vi "DAQ_CounterTrigger_DO_AO_2DAQ.vi"(8 "error in (no error)":errorcluster) -> (0 "error out":errorcluster)   [LabVIEW 2025]
uses:
  SubVIs/State_Machine_Ctrl.ctl
  <vilib>/DAQmx/write.llb/DAQmx Write (Digital 1D Wfm NChan NSamp).vi
  <vilib>/DAQmx/write.llb/DAQmx Write (Analog 1D Wfm NChan NSamp).vi
  <vilib>/Waveform/DWDTOps.llb/DWDT Uncompress Digital.vi
  <vilib>/DAQmx/miscellaneous.llb/DAQmx Fill In Error Info.vi
  <resource>/objmgr/daqmx.rc
panel:
  in  "Z":bool=TRUE
  in  "AO Z":tag="USB-6211/ao1"
  out "AO WF":waveform(dbl)[](graph)=[{"t0"=timestamp(0 s since 1904-01-01), "dt"=0.0001, "Y"=array[9000 elements]}, {"t0"=timestamp(0 s since 1904-01-01), "dt"=0.0001, "Y"=array[9000 elements]}, {"t0"=timestamp(0 s since 1904-01-01), "dt"=0.0001, "Y"=array[9000 elements]}, {"t0"=timestamp(0 s since 1904-01-01), "dt"=0.0001, "Y"=array[9000 elements]}]
  out "DO WF":digitalwaveform[](graph)=[{"t0"=timestamp(0 s since 1904-01-01), "dt"=0.0001, "Y"={"transitions"=[], "data"=array9000x1[9000 elements]}}, {"t0"=timestamp(0 s since 1904-01-01), "dt"=0.0001, "Y"={"transitions"=[], "data"=array9000x1[9000 elements]}}, {"t0"=timestamp(0 s since 1904-01-01), "dt"=0.0001, "Y"={"transitions"=[], "data"=array9000x1[9000 elements]}}, {"t0"=timestamp(0 s since 1904-01-01), "dt"=0.0001, "Y"={"transitions"=[], "data"=array9000x1[9000 elements]}}]
  in  "Polar | ON/OFF":bool=TRUE
  in  "AO | %":dbl[](array[slide])=[9.734513274336283, 23.008849557522126, 41.5929203539823, 65.48672566371681] min=0.0 max=100.0 step=1.0 scale=0.0..100.0
  in  "AO | ON/OFF":bool[](array[boolean])=[TRUE, TRUE, TRUE, TRUE]
  in  "AO Laser":tag="USB-6363/ao0:3"
  in  "AO pockels":tag="USB-6211/ao0"
  in  "DO | ON/OFF":bool[](array[boolean])=[TRUE, TRUE, TRUE, TRUE, TRUE]
  in  "Pre-activation time (s)":dbl=0.03
  in  "Start":bool
  in  "Timing source":tag="OnboardClock"
  in  "Readout time (s)":dbl=0.02
  in  "Exposure time (s)":dbl=0.05
  in  "DO | Trigger":tag="/USB-6363/PFI12"
  in  "DO":tag="USB-6363/port0/line0:4"
  in  "Counter":tag="USB-6363/ctr0"
  in  "Stop":bool
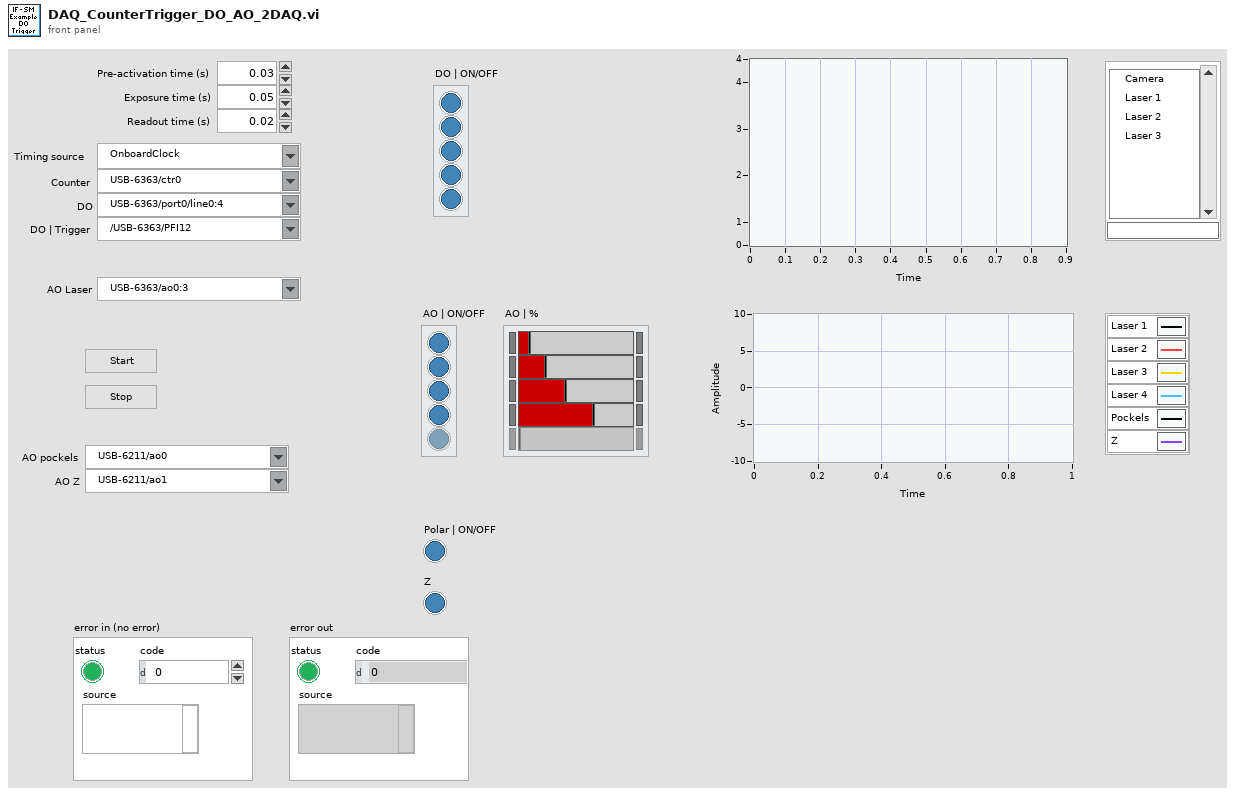
[diagram p1: front panel]
types:
  T1 = typedef "State_Machine_Ctrl.ctl" = enum16{"Initialize", "Wait for Event", "Setup_DAQ", "Create WF", "Generate WF", "Stop"}
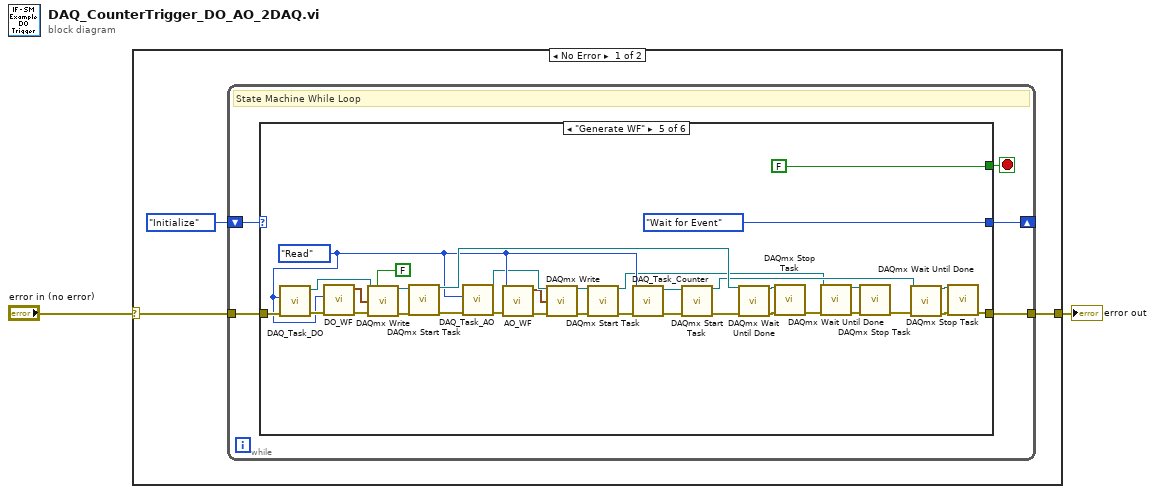
[diagram p0: block diagram]
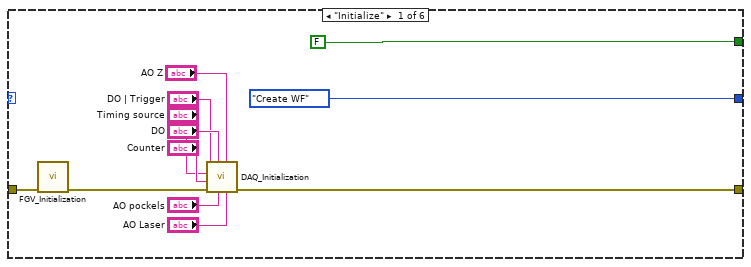
[diagram p2: hidden frame]
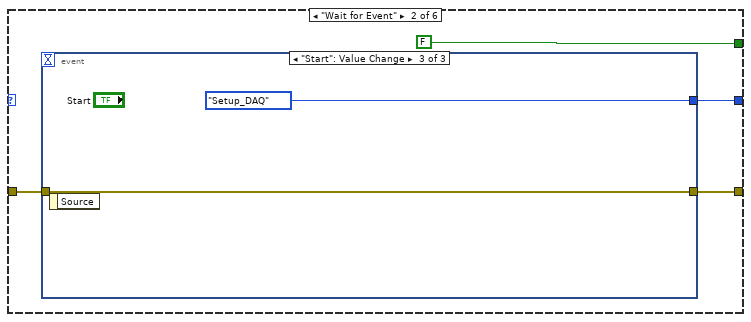
[diagram p3: hidden frame]
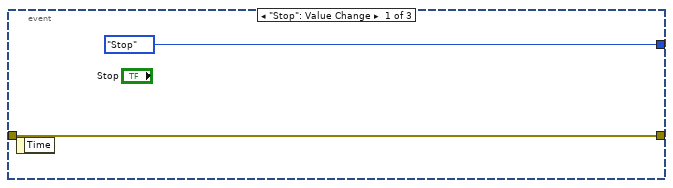
[diagram p4: hidden frame]
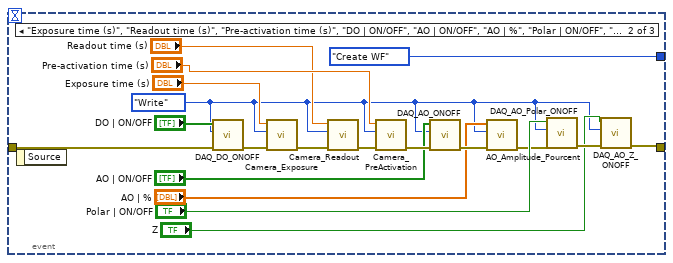
[diagram p5: hidden frame]
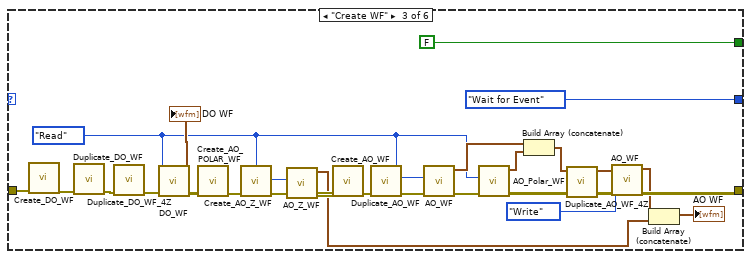
[diagram p6: hidden frame]
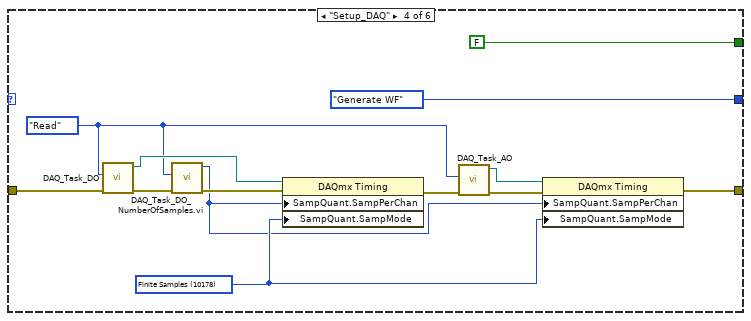
[diagram p7: hidden frame]
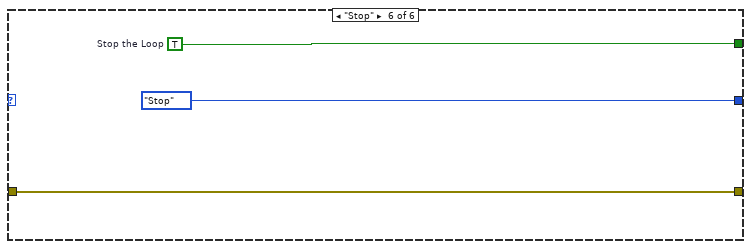
[diagram p8: hidden frame]
diagram:
  n1 = case shown="No Error" "error in (no error)" {
    selector: "error in (no error)" -> [w4 w126]
    tunnel: [w3 w126] -> w2
    frame No Error {
      n2 = while {
        shift-right: [w9] -> _
        shift-left: State_Machine_Ctrl."Initialize" ("Initial State") -> [w10]
        tunnel: w4 -> [w7]
        tunnel: [w6] -> w3
        stop <- w8 stop-if-true
        # "State Machine While Loop"
        n3 = case "State Machine Case Structure" shown="\"Generate WF\"" w10 {
          tunnel: [State_Machine_Ctrl."Create WF" ("Initial State") w26 State_Machine_Ctrl."Wait for Event" ("Initial State") State_Machine_Ctrl."Generate WF" ("Initial State") State_Machine_Ctrl."Wait for Event" ("Initial State") State_Machine_Ctrl."Stop" ("Initial State")] -> w9
          tunnel: [FALSE ("Stop the Loop") FALSE ("Stop the Loop") FALSE ("Stop the Loop") FALSE ("Stop the Loop") FALSE ("Stop the Loop") w125] -> w8
          tunnel: w7 -> [w20 w24 w73 w86 w119 w123]
          tunnel: [w21 w23 w54 w83 w106 w123] -> w6
          frame "Initialize" {
            # "Initialize - In this example, the only initialization required is to specify that the next state for the state machine is \"Wait for Event\"."
            n4 = call "FGV_Initialization.vi"("error in (no error)"=w20) -> ("error out"=w19:errorcluster)  [unwired: 10 in]
            n5 = call "DAQ_Initialization.vi"("AO Lasers"="AO Laser", "AO Z"="AO Z", "AO Pockels"="AO pockels", "DO"="DO", "error in (no error)"=w19, "Counter"="Counter", "Timing source"="Timing source", "DO | Trigger"="DO | Trigger") -> ("error out"=w21:errorcluster)  [unwired: 3 in]
          }
          frame "Wait for Event" {
            # "Wait for Event - An Event Structure is used to monitor the user interface for events. In each frame of the Event Structure, the next state of the state machine is specified based on which button was pressed."
            n6 = event shown="[2] \"Start\": Value Change" {
              selector: _ -> [_ _ _]
              dyn-events: _ -> [_ _ _]
              timeout: _ -> [_ _ _]
              tunnel: [State_Machine_Ctrl."Stop" ("Initial State") State_Machine_Ctrl."Create WF" ("Initial State") State_Machine_Ctrl."Setup_DAQ" ("Initial State")] -> w26
              tunnel: w24 -> [w27 w43 w48]
              tunnel: [w27 w31 w48] -> w23
              event "Stop": Value Change {
                n7 = event-data() -> ()  [unwired: 1 in, 1 out]
              }
              event "Exposure time (s)", "Readout time (s)", "Pre-activation time (s)", "DO | ON/OFF", "AO | ON/OFF", "AO | %", "Polar | ON/OFF", "Z": Value Change {
                w29 = enum16{"Write", "Read"}."Write" ("Action")
                n8 = event-data() -> ()  [unwired: 1 in, 1 out]
                n9 = call "DAQ_DO_ONOFF.vi"("error in"=w43, "Action"=w29, "DO | ON/OFF"="DO | ON/OFF") -> ("error out"=w46:errorcluster)  [unwired: 7 in, 1 out]
                n10 = call "Camera_Exposure.vi"("error in"=w46, "Action"=w29, "Exposure (s)"="Exposure time (s)") -> ("error out"=w45:errorcluster)  [unwired: 7 in, 1 out]
                n11 = call "Camera_Readout.vi"("error in"=w45, "Action"=w29, "Camera_Readout"="Readout time (s)") -> ("error out"=w44:errorcluster)  [unwired: 7 in, 1 out]
                n12 = call "Camera_PreActivation.vi"("error in"=w44, "Action"=w29, "Camera_PreActivation"="Pre-activation time (s)") -> ("error out"=w38:errorcluster)  [unwired: 7 in, 1 out]
                n13 = call "DAQ_AO_ONOFF.vi"("error in"=w38, "Action"=w29, "AO | ON/OFF"="AO | ON/OFF") -> ("error out"=w36:errorcluster)  [unwired: 7 in, 1 out]
                n14 = call "AO_Amplitude_Pourcent.vi"("error in"=w36, "Action"=w29, "AO | %"="AO | %") -> ("error out"=w33:errorcluster)  [unwired: 7 in, 1 out]
                n15 = call "DAQ_AO_Polar_ONOFF.vi"("error in"=w33, "Action"=w29, "ON / OFF"="Polar | ON/OFF") -> ("error out"=w32:errorcluster)  [unwired: 7 in, 1 out]
                n16 = call "DAQ_AO_Z_ONOFF.vi"("error in"=w32, "Action"=w29, "ON / OFF"="Z") -> ("error out"=w31:errorcluster)  [unwired: 7 in, 1 out]
              }
              event "Start": Value Change {
                n17 = event-data() -> ()  [unwired: 1 in, 1 out]
              }
            }
          }
          frame "Create WF" {
            w63 = enum16{"Write", "Read"}."Read" ("Action")
            n18 = call "Create_DO_WF.vi"("error in"=w73) -> ("error out"=w72:errorcluster)  [unwired: 10 in]
            n19 = call "Duplicate_DO_WF.vi"("error in"=w72) -> ("error out"=w60:errorcluster)  [unwired: 10 in]
            n20 = call "Duplicate_DO_WF_4Z.vi"("error in"=w60) -> ("error out"=w59:errorcluster)  [unwired: 10 in]
            n21 = call "DO_WF.vi"("error in"=w59, "Action"=w63) -> ("error out"=w58:errorcluster, "Digital WF"=→"DO WF":digitalwaveform[])  [unwired: 8 in]
            n22 = call "Create_AO_POLAR_WF.vi"("error in"=w58) -> ("error out"=w64:errorcluster)  [unwired: 10 in]
            n23 = call "Create_AO_Z_WF.vi"("error in"=w64) -> ("error out"=w62:errorcluster)  [unwired: 10 in]
            n24 = call "AO_Z_WF.vi"("error in"=w62, "Action"=w63) -> ("error out"=w61:errorcluster, "AO Z WF"=w52:waveform(dbl))  [unwired: 8 in]
            n25 = call "Create_AO_WF.vi"("error in"=w61) -> ("error out"=w70:errorcluster)  [unwired: 10 in]
            n26 = call "Duplicate_AO_WF.vi"("error in (no error)"=w70) -> ("error out"=w69:errorcluster)  [unwired: 10 in]
            n27 = call "AO_WF.vi"("error in"=w69, "Action"=w63) -> ("error out"=w71:errorcluster, "AO WF"=w66:waveform(dbl)[])  [unwired: 8 in]
            n28 = call "AO_Polar_WF.vi"("error in"=w71, "Action"=w63) -> ("error out"=w53:errorcluster, "AO Poalr WF"=w65:waveform(dbl))  [unwired: 8 in]
            n29 = Build Array (concatenate)(w66, w65) -> (w57:waveform(dbl)[])
            n30 = call "Duplicate_AO_WF_4Z.vi"("error in (no error)"=w53, "AO WF"=w57) -> ("error out"=w55:errorcluster, "AO WF 2"=w56:waveform(dbl)[])  [unwired: 8 in]
            n31 = call "AO_WF.vi"("error in"=w55, "Action"=enum16{"Write", "Read"}."Write", "AO WF"=w56) -> ("error out"=w54:errorcluster, "AO WF"=w51:waveform(dbl)[])  [unwired: 7 in]
            n32 = Build Array (concatenate)(w51, w52) -> (→"AO WF":waveform(dbl)[])
          }
          frame "Setup_DAQ" {
            w80 = 10178 items=["Finite Samples"=10178, "Continuous Samples"=10123, "Hardware Timed Single Point"=12522] ("SampQuant.SampMode")
            w79 = enum16{"Write", "Read"}."Read" ("Action")
            n33 = call "DAQ_Task_DO.vi"("error in"=w86, "Action"=w79) -> ("error out"=w78:errorcluster, "DAQ_Task_DO"=w85:refnum<k21>)  [unwired: 8 in]
            n34 = call "DAQ_Task_DO_NumberOfSamples.vi.vi"("error in"=w78, "Action"=w79) -> ("error out"=w77:errorcluster, "Samples"=w76:u32)  [unwired: 8 in]
            n35 = property class="DAQmx Timing"(reference=w85, error in=w77, "SampQuant.SampPerChan"=w76, "SampQuant.SampMode"=w80) -> (error out=w81:errorcluster)  [unwired: 1 out]
            n36 = call "DAQ_Task_AO.vi"("error in"=w81, "Action"=w79) -> ("error out"=w84:errorcluster, "DAQ_Task_DO"=w82:refnum<k21>)  [unwired: 8 in]
            n37 = property class="DAQmx Timing"(reference=w82, error in=w84, "SampQuant.SampPerChan"=w76, "SampQuant.SampMode"=w80) -> (error out=w83:errorcluster)  [unwired: 1 out]
          }
          frame "Generate WF" {
            w96 = enum16{"Write", "Read"}."Read" ("Action")
            n38 = call "DAQ_Task_DO.vi"("error in"=w119, "Action"=w96) -> ("error out"=w103:errorcluster, "DAQ_Task_DO"=w118:refnum<k21>)  [unwired: 8 in]
            n39 = call "DO_WF.vi"("error in"=w103, "Action"=w96) -> ("error out"=w102:errorcluster, "Digital WF"=w104:digitalwaveform[])  [unwired: 8 in]
            n40 = call-poly <vilib>:"DAQmx Write.vi"("task/channels in"=w118, "auto start"=FALSE, "data"=w104, "error in"=w102) -> ("task out"=w117:refnum<k21>, "error out"=w120:errorcluster)  [unwired: 9 in, 1 out]
            n41 = call <vilib>:"DAQmx Start Task.vi"("task/channels in"=w117, "error in"=w120) -> ("task out"=w110:refnum<k21>, "error out"=w105:errorcluster)  [unwired: 12 in]
            n42 = call "DAQ_Task_AO.vi"("error in"=w105, "Action"=w96) -> ("error out"=w97:errorcluster, "DAQ_Task_DO"=w95:refnum<k21>)  [unwired: 8 in]
            n43 = call "AO_WF.vi"("error in"=w97, "Action"=w96) -> ("error out"=w93:errorcluster, "AO WF"=w94:waveform(dbl)[])  [unwired: 8 in]
            n44 = call-poly <vilib>:"DAQmx Write.vi"("task/channels in"=w95, "data"=w94, "error in"=w93) -> ("task out"=w92:refnum<k21>, "error out"=w91:errorcluster)  [unwired: 10 in, 1 out]
            n45 = call <vilib>:"DAQmx Start Task.vi"("task/channels in"=w92, "error in"=w91) -> ("task out"=w89:refnum<k21>, "error out"=w90:errorcluster)  [unwired: 12 in]
            n46 = call "DAQ_Task_Counter.vi"("error in"=w90, "Action"=w96) -> ("error out"=w115:errorcluster, "DAQ_Task_Counter"=w116:refnum<k21>)  [unwired: 8 in]
            n47 = call <vilib>:"DAQmx Start Task.vi"("task/channels in"=w116, "error in"=w115) -> ("task out"=w108:refnum<k21>, "error out"=w107:errorcluster)  [unwired: 12 in]
            n48 = call <vilib>:"DAQmx Wait Until Done.vi"("task/channels in"=w110, "error in"=w107) -> ("task out"=w109:refnum<k21>, "error out"=w111:errorcluster)  [unwired: 12 in]
            n49 = call <vilib>:"DAQmx Stop Task.vi"("task/channels in"=w109, "error in"=w111) -> ("error out"=w100:errorcluster)  [unwired: 12 in, 1 out]
            n50 = call <vilib>:"DAQmx Wait Until Done.vi"("task/channels in"=w89, "error in"=w100) -> ("task out"=w98:refnum<k21>, "error out"=w101:errorcluster)  [unwired: 12 in]
            n51 = call <vilib>:"DAQmx Stop Task.vi"("task/channels in"=w98, "error in"=w101) -> ("error out"=w99:errorcluster)  [unwired: 12 in, 1 out]
            n52 = call <vilib>:"DAQmx Wait Until Done.vi"("task/channels in"=w108, "error in"=w99) -> ("task out"=w113:refnum<k21>, "error out"=w112:errorcluster)  [unwired: 12 in]
            n53 = call <vilib>:"DAQmx Stop Task.vi"("task/channels in"=w113, "error in"=w112) -> ("error out"=w106:errorcluster)  [unwired: 12 in, 1 out]
          }
          frame "Stop" {
            w125 = TRUE  # Stop the Loop
            # "Stop - Stop the VI. This is the only state that specifies a TRUE value for the loop conditional terminal."
          }
        }
      }
    }
    frame Error {
    }
  }
  "error out" <- w2
